vi "Signal_acquisition_v1.vi"() -> ()   [LabVIEW 2015]
uses:
  <vilib>/measure/matone.llb/Extract Single Tone Information 1 Chan.vi
  <vilib>/measure/madcrms.llb/Basic Averaged DC-RMS for 1 Chan.vi
  <vilib>/measure/NI_MAPro.lvlib
  <vilib>/Analysis/NI_AALPro.lvlib
panel:
  out "Time Shift":dbl
  out "magnitude":dbl
  out "Freq":dbl=0.3
  out "Phase Shift":dbl
  in  "SAVE DATA":bool
  out "AMPLITUDE\nRESULT":dbl
  out "REFERENCE amplitude":dbl format="%.2p"
  out "output \ndetected \namplitude":dbl[](array[numeric])
  in  "MEASURE AMPLITUD":bool
  in  "MEASURE PHASE":bool
  out "Phase":dbl(knob) scale=0.0..90.0
  out "detected \nphase (deg) 2":dbl format="%.2p"
  out "detected \nfrequency 2":dbl format="%.2p"
  out "DC value 2":dbl format="%0.2p"
  in  "input 2":u16
  in  "timeout ms (2000) 2":i32=2000
  out "REAL TIME MEASUREMENT":dbl[](graph)
  in  "Trigger Mode 2":string(combo)="CH2_NE"
  in  "Pause for buffer (ms) 2":u32=100
  in  "MEASURE REFERENCE":bool
  out "detected phase (deg)":dbl format="%.2p"
  out "detected frequency":dbl format="%.2p"
  out "MEASURED amplitud":dbl format="%.2p"
  out "DC value":dbl format="%0.2p"
  in  "input 1":u16
  out "Acquisition time complete":u32
  out "millisecond final timer":u32
  out "millisecond begin timer":u32
  out "millisecond timer value":u32
  out "Numeric":i32
  in  "timeout ms\n (2000)":i32=2000
  in  "timeout ms\n (2000)":i32=2000
  in  "timeout ms\n (2000)":i32=2000
  in  "?":bool
  out "error out":errorcluster
  out "WAVEFORM BASE LINE":dbl[](graph)
  in  "Trigger Mode":string(combo)="CH2_NE"
  in  "Pause for\n buffer (ms)":u32=100
  in  "Delay\n (# Samples)":i32 max=16348
  in  "Trigger Level \n(0 mV)":i32
  in  "IP address":string="161.111.10.6"
  in  "Decimation":u16(ring)=8 items=["65536"=65535, "8192"=8192, "1024"=1024, "64"=64, "8"=8, "1"=1]
  in  "error in":errorcluster
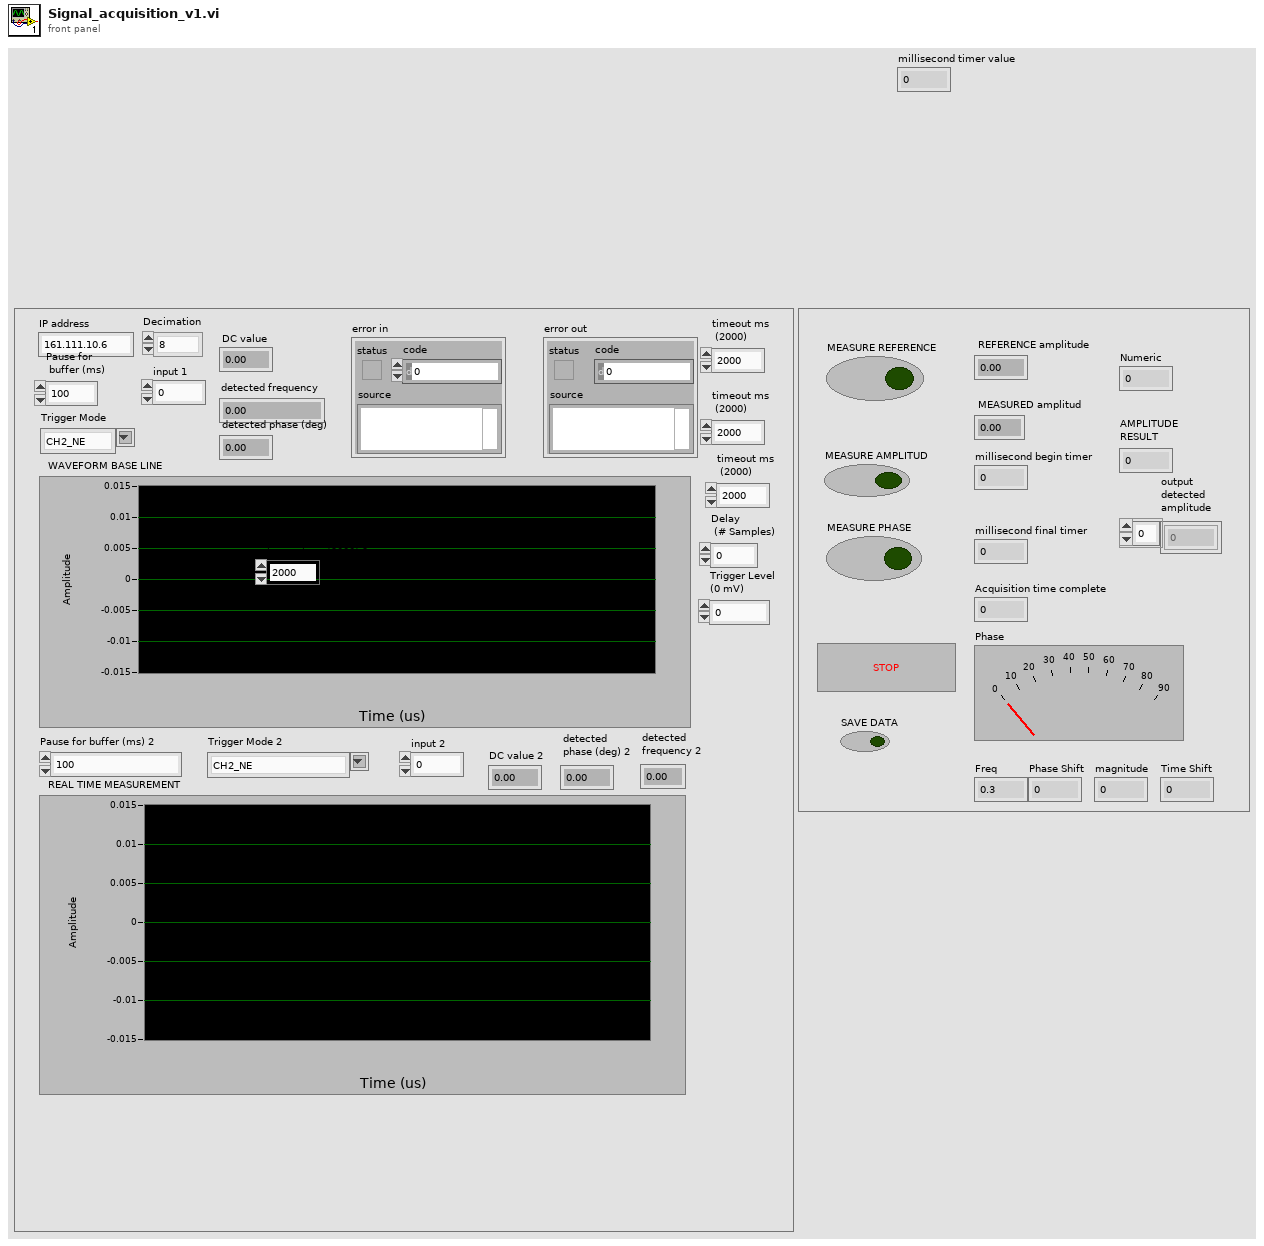
[diagram p1: front panel]
types:
  T1 = enum16{"Standard", "Buffered", "CRLF", "Immediate"}
  T2 = enum32{"none", "input signal", "detected signal", "residual signal"}
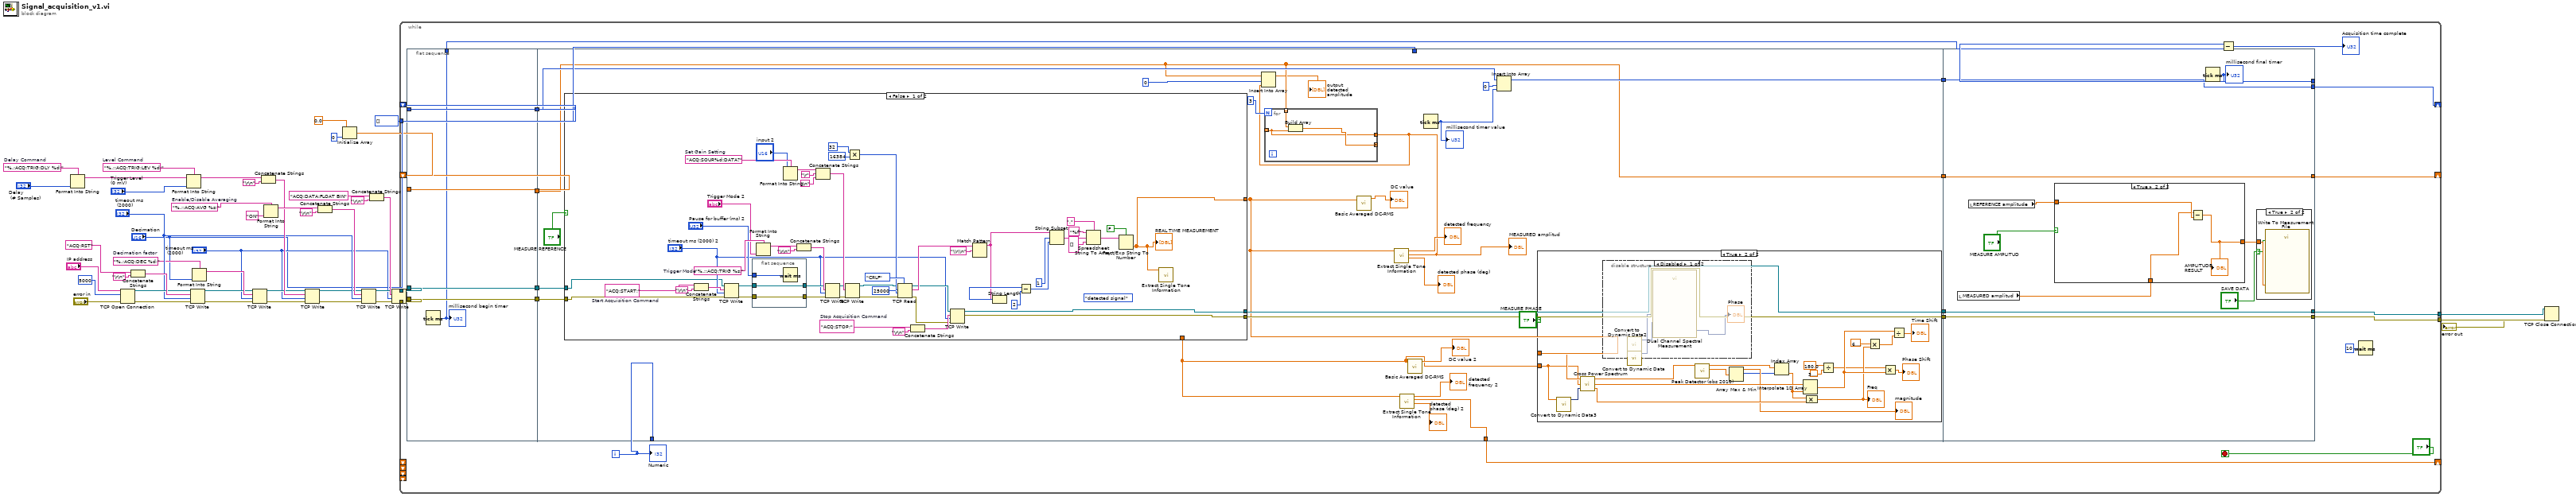
[diagram p0: block diagram]
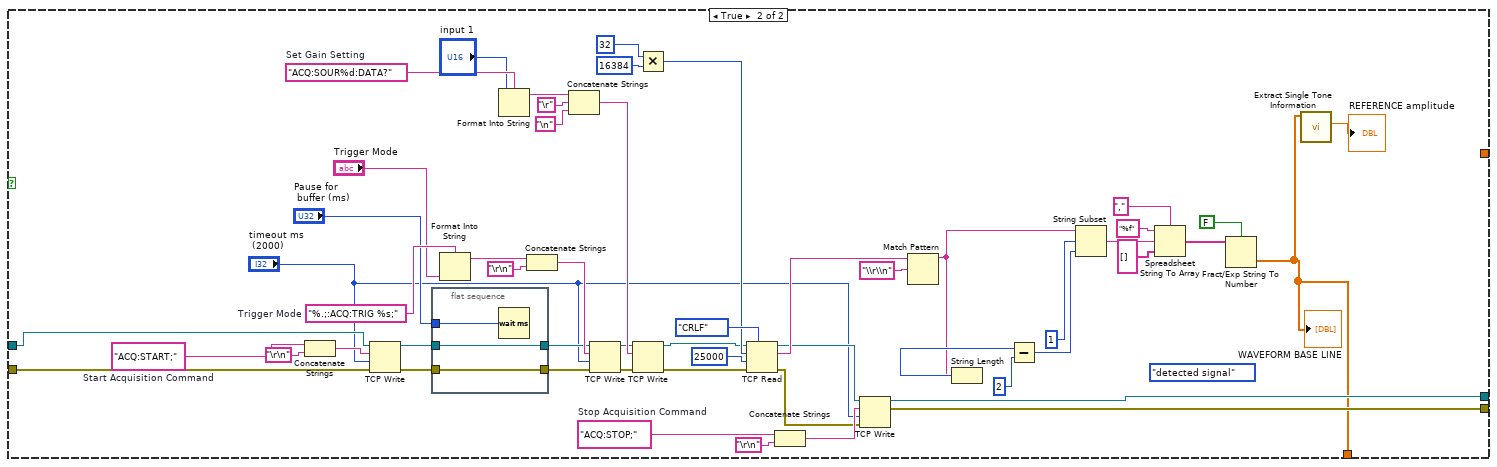
[diagram p4: hidden frame]
diagram:
  w12 = "%.;:ACQ:AVG %s;"  # Enable/Disable Averaging
  w20 = "%.;ACQ:DEC %d;"  # Decimation factor
  w21 = "%.;ACQ:TRIG:DLY %d;"  # Delay Command
  w22 = "%.;:ACQ:TRIG:LEV %d;"  # Level Command
  n1 = Format Into String(format string=w21, "Delay\n (# Samples)") -> (resulting string=w40:string)  [unwired: 2 in, 1 out]
  n2 = TCP Open Connection(address="IP address", remote port or service name=u16 5000, error in (no error)="error in") -> (connection ID=w34:refnum<k5>, error out=w33:errorcluster)  [unwired: 2 in]
  n3 = Concatenate Strings("ACQ:RST" ("SCPI Message"), "\r\n") -> (w36:string)
  n4 = Format Into String(format string=w22, initial string=w40, "Trigger Level \n(0 mV)") -> (resulting string=w37:string)  [unwired: 1 in, 1 out]
  n5 = TCP Write(connection ID=w34, data in=w36, error in (no error)=w33, 9:"timeout ms\n (2000)") -> (connection ID out=w18:refnum<k5>, error out=w17:errorcluster)  [unwired: 1 out]
  n6 = Format Into String(format string=w20, "Decimation") -> (resulting string=w19:string)  [unwired: 2 in, 1 out]
  n7 = TCP Write(connection ID=w18, data in=w19, error in (no error)=w17, 9:"timeout ms\n (2000)") -> (connection ID out=w16:refnum<k5>, error out=w15:errorcluster)  [unwired: 1 out]
  n8 = Concatenate Strings(w37, "\r\n") -> (w31:string)
  n9 = Format Into String(format string=w12, "ON") -> (resulting string=w43:string)  [unwired: 2 in, 1 out]
  n10 = TCP Write(connection ID=w16, data in=w31, error in (no error)=w15, 9:"timeout ms\n (2000)") -> (connection ID out=w14:refnum<k5>, error out=w13:errorcluster)  [unwired: 1 out]
  n11 = Concatenate Strings(w43, "\r\n") -> (w32:string)
  n12 = Initialize Array(0.0 ("element"), 0 ("dimension size")) -> (w1:dbl[])
  n13 = TCP Write(connection ID=w14, data in=w32, error in (no error)=w13, 9:"timeout ms\n (2000)") -> (connection ID out=w10:refnum<k5>, error out=w9:errorcluster)  [unwired: 1 out]
  n14 = Concatenate Strings("ACQ:DATA:FLOAT BIN" ("SCPI Message"), "\r\n") -> (w28:string)
  n15 = TCP Write(connection ID=w10, data in=w28, error in (no error)=w9, 9:"timeout ms\n (2000)") -> (connection ID out=w7:refnum<k5>, error out=w6:errorcluster)  [unwired: 1 out]
  n16 = while {
    tunnel: w7 -> [w70]
    tunnel: [w65] -> w27
    tunnel: [w64] -> w26
    tunnel: w6 -> [w68]
    shift-right: [w67] -> _
    shift-left: u32[] [] -> [w66]
    tunnel: "Decimation" -> [w54]
    shift-right: [w51] -> _
    shift-left: w1 -> [w48]
    shift-right: [w47] -> _
    shift-left: _ -> [_]
    shift-left: _ -> [_]
    shift-left: _ -> [_]
    shift-left: _ -> [_]
    i -> [w50]
    stop <- "?" stop-if-true
    n17 = flat-sequence {
      tunnel: w66 -> [w73]
      tunnel: w68 -> [w74]
      tunnel: w70 -> [w75]
      tunnel: [w75] -> w60
      tunnel: [w74] -> w59
      tunnel: [w73] -> w58
      tunnel: [w72] -> w56
      tunnel: [w71] -> w49
      tunnel: w48 -> [w71]
      tunnel: [w95] -> w63
      tunnel: [w93] -> w62
      tunnel: [w92] -> w61
      tunnel: w60 -> [w99]
      tunnel: w59 -> [w98]
      tunnel: w58 -> [w94]
      tunnel: w54 -> [_]
      tunnel: [w87] -> w52
      tunnel: w50 -> [_]
      tunnel: w49 -> [w87]
      tunnel: [w76] -> w47
      tunnel: [w244] -> w64
      tunnel: [w245] -> w65
      tunnel: [w246] -> w67
      tunnel: w63 -> [w246]
      tunnel: w62 -> [w245]
      tunnel: w61 -> [w244]
      tunnel: [w243] -> w57
      tunnel: w52 -> [w242]
      tunnel: [w242] -> w51
      frame #0 {
        n18 = Tick Count (ms)() -> (millisecond timer value=w72:u32)
        "millisecond begin timer" <- w72
      }
      frame #1 {
        n19 = case shown="False" "MEASURE REFERENCE" {
          tunnel: w99 -> [w124 w227]
          tunnel: w98 -> [w127 w191]
          tunnel: [w125 w188] -> w93
          tunnel: [w126 w183] -> w92
          tunnel: [w123 _] -> w79
          tunnel: [_ w179] -> w81
          frame False {
            w134 = "ACQ:STOP;"  # Stop Acquisition Command
            (unwired) T2."detected signal" ("export mode")
            w144 = "ACQ:SOUR%d:DATA?"  # Set Gain Setting
            w171 = "%.;:ACQ:TRIG %s;"  # Trigger Mode
            w173 = "ACQ:START;"  # Start Acquisition Command
            n20 = Concatenate Strings(w173, "\r\n") -> (w174:string)
            n21 = TCP Write(connection ID=w124, data in=w174, error in (no error)=w127, 9:"timeout ms (2000) 2") -> (connection ID out=w148:refnum<k5>, error out=w147:errorcluster)  [unwired: 1 out]
            n22 = flat-sequence {
              tunnel: "Pause for buffer (ms) 2" -> [w177]
              tunnel: [w176] -> w146
              tunnel: [w175] -> w145
              tunnel: w148 -> [w176]
              tunnel: w147 -> [w175]
              frame #0 {
                n23 = Wait (ms)(milliseconds to wait=w177) -> ()  [unwired: 1 out]
              }
            }
            n24 = Format Into String(format string=w171, "Trigger Mode 2") -> (resulting string=w168:string)  [unwired: 2 in, 1 out]
            n25 = Format Into String(format string=w144, "input 2") -> (resulting string=w142:string)  [unwired: 2 in, 1 out]
            n26 = Concatenate Strings(w168, "\r\n") -> (w169:string)
            n27 = Concatenate Strings(w142, "\r", "\n") -> (w141:string)
            n28 = TCP Write(connection ID=w146, data in=w169, error in (no error)=w145, 9:"timeout ms (2000) 2") -> (connection ID out=w139:refnum<k5>, error out=w138:errorcluster)  [unwired: 1 out]
            n29 = TCP Write(connection ID=w139, data in=w141, error in (no error)=w138) -> (connection ID out=w140:refnum<k5>, error out=w137:errorcluster)  [unwired: 1 in, 1 out]
            n30 = Multiply(x=32, y=16384 ("bytes to read")) -> (x*y=w149:i32)
            n31 = TCP Read(connection ID=w140, bytes to read=w149, error in (no error)=w137, 7:T1."CRLF" ("mode (standard)"), 9:25000 ("timeout ms (25000)")) -> (connection ID out=w135:refnum<k5>, data out=w150:string, error out=w131:errorcluster)
            n32 = Concatenate Strings(w134, "\r\n") -> (w132:string)
            n33 = TCP Write(connection ID=w135, data in=w132, error in (no error)=w131, 9:"timeout ms (2000) 2") -> (connection ID out=w125:refnum<k5>, error out=w126:errorcluster)  [unwired: 1 out]
            n34 = Match Pattern(string=w150, regular expression="\\r\\n") -> (before substring=w156:string)  [unwired: 1 in, 3 out]
            n35 = String Length(string=w156) -> (length=w159:i32)
            n36 = Subtract(x=w159, y=2) -> (x-y=w160:i32)
            n37 = String Subset(string=w156, offset (0)=1, length (rest)=w160) -> (substring=w157:string)
            n38 = Spreadsheet String To Array(delimiter (Tab)=",", format string="%f", spreadsheet string=w157, array type (2D Dbl)=string[] [] ("Array")) -> (array=w163:string[])
            n39 = Fract/Exp String To Number(use system decimal point (T)=FALSE, string=w163) -> (number=w123:dbl[])  [unwired: 3 out]
            "REAL TIME MEASUREMENT" <- w123
            n40 = call-poly <vilib>:"Extract Single Tone Information.vi"("time signal in"=w123) -> ()  [unwired: 5 in, 6 out]
          }
          frame True {
            w187 = "ACQ:STOP;"  # Stop Acquisition Command
            (unwired) T2."detected signal" ("export mode")
            w199 = "ACQ:SOUR%d:DATA?"  # Set Gain Setting
            w226 = "%.;:ACQ:TRIG %s;"  # Trigger Mode
            w229 = "ACQ:START;"  # Start Acquisition Command
            n41 = Concatenate Strings(w229, "\r\n") -> (w230:string)
            n42 = TCP Write(connection ID=w227, data in=w230, error in (no error)=w191, 9:"timeout ms\n (2000)") -> (connection ID out=w203:refnum<k5>, error out=w202:errorcluster)  [unwired: 1 out]
            n43 = flat-sequence {
              tunnel: "Pause for\n buffer (ms)" -> [w233]
              tunnel: [w232] -> w201
              tunnel: [w231] -> w200
              tunnel: w203 -> [w232]
              tunnel: w202 -> [w231]
              frame #0 {
                n44 = Wait (ms)(milliseconds to wait=w233) -> ()  [unwired: 1 out]
              }
            }
            n45 = Format Into String(format string=w226, "Trigger Mode") -> (resulting string=w223:string)  [unwired: 2 in, 1 out]
            n46 = Format Into String(format string=w199, "input 1") -> (resulting string=w197:string)  [unwired: 2 in, 1 out]
            n47 = Concatenate Strings(w223, "\r\n") -> (w224:string)
            n48 = Concatenate Strings(w197, "\r", "\n") -> (w196:string)
            n49 = TCP Write(connection ID=w201, data in=w224, error in (no error)=w200, 9:"timeout ms\n (2000)") -> (connection ID out=w194:refnum<k5>, error out=w193:errorcluster)  [unwired: 1 out]
            n50 = TCP Write(connection ID=w194, data in=w196, error in (no error)=w193) -> (connection ID out=w195:refnum<k5>, error out=w192:errorcluster)  [unwired: 1 in, 1 out]
            n51 = Multiply(x=32, y=16384 ("bytes to read")) -> (x*y=w204:i32)
            n52 = TCP Read(connection ID=w195, bytes to read=w204, error in (no error)=w192, 7:T1."CRLF" ("mode (standard)"), 9:25000 ("timeout ms (25000)")) -> (connection ID out=w189:refnum<k5>, data out=w205:string, error out=w184:errorcluster)
            n53 = Concatenate Strings(w187, "\r\n") -> (w185:string)
            n54 = TCP Write(connection ID=w189, data in=w185, error in (no error)=w184, 9:"timeout ms\n (2000)") -> (connection ID out=w188:refnum<k5>, error out=w183:errorcluster)  [unwired: 1 out]
            n55 = Match Pattern(string=w205, regular expression="\\r\\n") -> (before substring=w211:string)  [unwired: 1 in, 3 out]
            n56 = String Length(string=w211) -> (length=w214:i32)
            n57 = Subtract(x=w214, y=2) -> (x-y=w215:i32)
            n58 = String Subset(string=w211, offset (0)=1, length (rest)=w215) -> (substring=w212:string)
            n59 = Spreadsheet String To Array(delimiter (Tab)=",", format string="%f", spreadsheet string=w212, array type (2D Dbl)=string[] [] ("Array")) -> (array=w218:string[])
            n60 = Fract/Exp String To Number(use system decimal point (T)=FALSE, string=w218) -> (number=w179:dbl[])  [unwired: 3 out]
            "WAVEFORM BASE LINE" <- w179
            n61 = call-poly <vilib>:"Extract Single Tone Information.vi"("time signal in"=w179) -> ("detected amplitude"=→"REFERENCE amplitude":dbl)  [unwired: 5 in, 5 out]
          }
        }
        n62 = call-poly <vilib>:"Basic Averaged DC-RMS.vi"("signal in"=w79) -> ("DC value"=→"DC value":dbl)  [unwired: 7 in, 3 out]
        n63 = call-poly <vilib>:"Extract Single Tone Information.vi"("time signal in"=w79) -> ("detected phase (deg)"=→"detected phase (deg)":dbl, "detected amplitude"=w78:dbl, "detected frequency"=→"detected frequency":dbl)  [unwired: 5 in, 3 out]
        "MEASURED amplitud" <- w78
        n64 = Insert Into Array(array=w87, index=0, new element=w78) -> (→"output \ndetected \namplitude":dbl[])
        n65 = for {
          N: 3 -> [_]
          tunnel: [w234] -> _ mode=indexing
          tunnel: w87 -> [w236] mode=indexing
          tunnel: [w235] -> _ mode=concatenating
          tunnel: w78 -> [w234]
          n66 = Build Array(w236, w234) -> (w235:dbl[])
        }
        n67 = call-poly <vilib>:"Extract Single Tone Information.vi"("time signal in"=w81) -> ("detected phase (deg)"=→"detected \nphase (deg) 2":dbl, "detected amplitude"=w76:dbl, "detected frequency"=→"detected \nfrequency 2":dbl)  [unwired: 5 in, 3 out]
        n68 = call-poly <vilib>:"Basic Averaged DC-RMS.vi"("signal in"=w81) -> ("DC value"=→"DC value 2":dbl)  [unwired: 7 in, 3 out]
        n69 = Tick Count (ms)() -> (millisecond timer value=w96:u32)
        "millisecond timer value" <- w96
        n70 = Insert Into Array(array=w94, index=0, new element=w96) -> (w95:u32[])
        n71 = case shown="True" "MEASURE PHASE" {
          tunnel: w79 -> [_ w102]
          tunnel: w81 -> [_ w100]
          frame False {
          }
          frame True {
            n72 = call "Convert to Dynamic Data3"("Array"=w100) -> ("Dynamic Data Type"=w101:dynamicdata)  [unwired: 3 in]
            n73 = call <vilib>:"Cross Power Spectrum.vi"("dt"=w101, "Signal Y (V)"=w100, "Signal X (V)"=w102) -> ("df"=w116:dbl, "Cross Power XY Spectrum Phase (radians)"=w117:dbl[], "Cross Power XY Spectrum Mag (V^2rms)"=w115:dbl[])
            n74 = disable-structure shown="Disabled" {
              frame Disabled {
                n75 = call "Convert to Dynamic Data2"() -> ("Dynamic Data Type"=w120:dynamicdata)  [unwired: 4 in]
                n76 = call "Convert to Dynamic Data"() -> ("Dynamic Data Type"=w122:dynamicdata)  [unwired: 4 in]
                n77 = call "Dual Channel Spectral Measurement"("Input Signal B"=w120, "Input Signal A"=w122) -> ("Phase"=→"Phase":dynamicdata)  [unwired: 8 in, 1 out]
              }
              frame Enabled {
              }
            }
            n78 = call <vilib>:"Peak Detector (obs 2010).vi"("X"=w115) -> ("Amplitudes"=w105:dbl[], "Locations"=w114:dbl[])  [unwired: 6 in, 3 out]
            n79 = Array Max & Min(array=w105) -> (max value=→"magnitude":dbl, max index (indices)=w104:i32)  [unwired: 2 out]
            n80 = Index Array(array=w114, index=w104) -> (element=w103:dbl)
            n81 = Interpolate 1D Array(1:w103, 2:w117) -> (0:w112:dbl)
            n82 = Compound Arithmetic op=MULTIPLY(w103, w116) -> (w110:dbl)
            "Freq" <- w110
            n83 = Divide(x=180.0, y=3.141592653589793) -> (x/y=w106:dbl)
            n84 = Multiply(x=6.283185307179586, y=w110) -> (x*y=w109:dbl)
            n85 = Multiply(x=w106, y=w112) -> (x*y=→"Phase Shift":dbl)
            n86 = Divide(x=w112, y=w109) -> (x/y=→"Time Shift":dbl)
          }
        }
      }
      frame #2 {
        n87 = local read "MEASURED amplitud"() -> (w240:dbl)
        n88 = local read "REFERENCE amplitude"() -> (w241:dbl)
        n89 = case shown="True" "MEASURE AMPLITUD" {
          tunnel: w241 -> [w249 w251]
          tunnel: w240 -> [_ w250]
          tunnel: [w249 w252] -> w238
          frame False {
          }
          frame True {
            n90 = Subtract(x=w250, y=w251) -> (x-y=w252:dbl)
            "AMPLITUDE\nRESULT" <- w252
          }
        }
        n91 = Tick Count (ms)() -> (millisecond timer value=w243:u32)
        "millisecond final timer" <- w243
        n92 = case shown="True" "SAVE DATA" {
          selector: "SAVE DATA" -> [_ w247]
          tunnel: w238 -> [_ w248]
          frame False {
          }
          frame True {
            n93 = call "Write To Measurement File"("Signals"=w248, "Enable"=w247) -> ()  [unwired: 15 in, 3 out]
          }
        }
      }
    }
    n94 = Subtract(x=w57, y=w56) -> (x-y=→"Acquisition time complete":u32)
    n95 = Wait (ms)(milliseconds to wait=u32 10) -> ()  [unwired: 1 out]
    "Numeric" <- w50
  }
  n96 = TCP Close Connection(connection ID=w27, error in (no error)=w26) -> (error out=→"error out":errorcluster)  [unwired: 1 in, 1 out]
